vi "FT10_Log Notifier.vi"(7 "Selector":T1, 8 "error in (no error)":errorcluster) -> (0 "error out":errorcluster, 3 "Notifier out":refnum<notifier>)   [LabVIEW 2015]
uses:
  Controls/Config_Log Notifier Enum.ctl
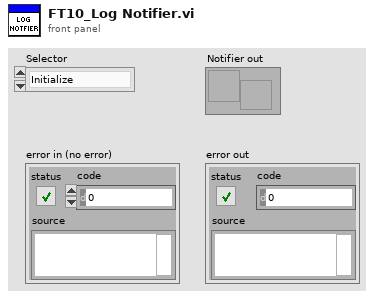
[diagram p1: front panel]
types:
  T1 = typedef "Config_Log Notifier Enum.ctl" = enum16{"Initialize", "Read Notifier", "Notify - True", "Notify - False", "Close"}
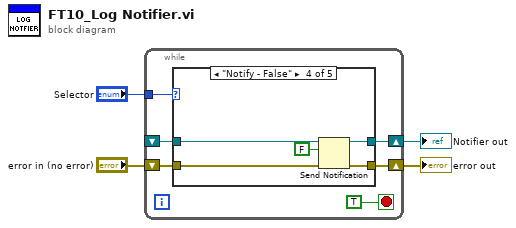
[diagram p0: block diagram]
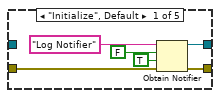
[diagram p2: hidden frame]
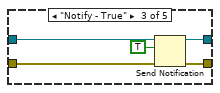
[diagram p4: hidden frame]
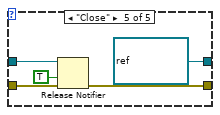
[diagram p5: hidden frame]
diagram:
  n1 = while {
    tunnel: "Selector" -> [w9]
    shift-right: [w6] -> w4
    shift-left: _ -> [w5]
    shift-right: [w7] -> w3
    shift-left: "error in (no error)" -> [w8]
    stop <- TRUE stop-if-true
    n2 = case shown="\"Notify - False\"" w9 {
      tunnel: w8 -> [w13 w17 w23 w28 w32]
      tunnel: [w12 w17 w22 w27 w31] -> w7
      tunnel: [w11 w18 w21 w26 refnum<notifier> refnum ("notifier out")] -> w6
      tunnel: w5 -> [_ w18 w20 w25 w33]
      frame "Initialize", Default {
        n3 = Obtain Notifier(name (unnamed)="Log Notifier", notification data type=FALSE, create if not found? (T)=TRUE, error in (no error)=w13) -> (notifier out=w11:refnum<notifier>, error out=w12:errorcluster)  [unwired: 1 out]
      }
      frame "Read Notifier" {
      }
      frame "Notify - True" {
        n4 = Send Notification(notification=TRUE, notifier=w20, error in (no error)=w23) -> (notifier out=w21:refnum<notifier>, error out=w22:errorcluster)
      }
      frame "Notify - False" {
        n5 = Send Notification(notification=FALSE, notifier=w25, error in (no error)=w28) -> (notifier out=w26:refnum<notifier>, error out=w27:errorcluster)
      }
      frame "Close" {
        n6 = Release Notifier(notifier=w33, force destroy? (F)=TRUE, error in (no error)=w32) -> (error out=w31:errorcluster)  [unwired: 2 out]
      }
    }
  }
  "error out" <- w3
  "Notifier out" <- w4
